vi "Find Transition.vi"(0 "State in":refnum<class "State.lvclass">, 5 "Target":string, 7 "Event":string, 9 "Type":string, 11 "error in (no error)":errorcluster) -> (4 "State thru":refnum<class "State.lvclass">, 6 "transIndex":i32, 8 "termination":bool, 15 "error out":errorcluster)   [LabVIEW 2015, in "State.lvclass"]
uses:
  State.lvclass
  Typedefs/Tosca-Event Type.ctl
  State.lvclass/State.ctl
  Termination/Termination.lvclass/Termination.ctl
  Timeout/Timeout.lvclass/Timeout.ctl
  Termination/Read Link to.vi
  Termination/Read Source.vi
  Termination/Read Type.vi
  Timeout/Read Link to.vi
  Timeout/Read Type.vi
  Timeout/Timeout.lvclass
  Termination/Termination.lvclass
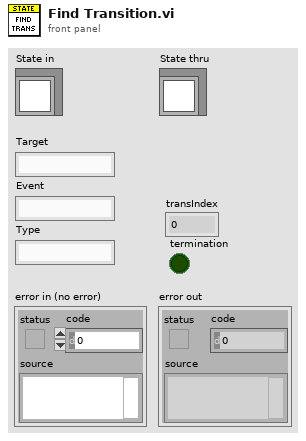
[diagram p1: front panel]
types:
  T1 = typedef "Tosca-Event Type.ctl" = enum16{"Normal", "CS+", "CS-"}
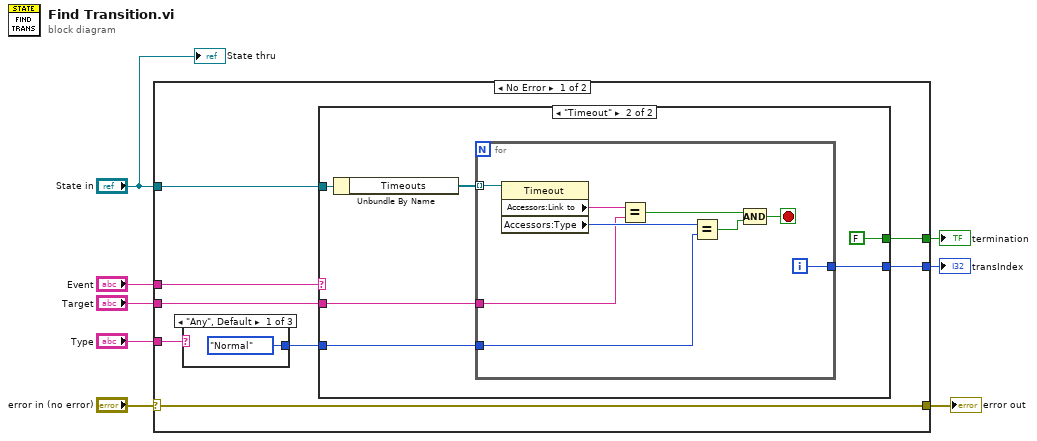
[diagram p0: block diagram]
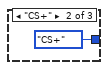
[diagram p2: hidden frame]
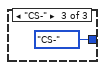
[diagram p3: hidden frame]
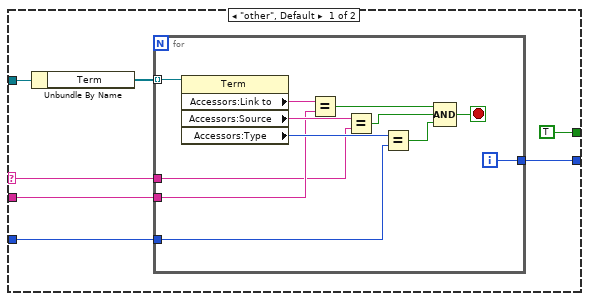
[diagram p4: hidden frame]
diagram:
  n1 = case shown="No Error" "error in (no error)" {
    selector: "error in (no error)" -> [w16 w54]
    tunnel: [w16 w54] -> w7
    tunnel: "State in" -> [w14 _]
    tunnel: "Type" -> [w10 _]
    tunnel: "Event" -> [w15 _]
    tunnel: "Target" -> [w13 _]
    tunnel: [w12 _] -> w3
    tunnel: [w11 _] -> w2
    frame No Error {
      n2 = case shown="\"Any\", Default" w10 {
        tunnel: [Tosca-Event_Type."Normal" ("Serialized.Type") Tosca-Event_Type."CS+" ("Serialized.Type") Tosca-Event_Type."CS-" ("Serialized.Type")] -> w9
        frame "Any", Default {
        }
        frame "CS+" {
        }
        frame "CS-" {
        }
      }
      n3 = case shown="\"Timeout\"" w15 {
        selector: w15 -> [w23 _]
        tunnel: w14 -> [w26 w44]
        tunnel: w13 -> [w24 w42]
        tunnel: [w22 w41] -> w12
        tunnel: [TRUE FALSE] -> w11
        tunnel: w9 -> [w20 w39]
        frame "other", Default {
          n4 = Unbundle By Name(w26) -> ("Term"=w25:refnum<class "Termination.lvclass">[])
          n5 = for {
            tunnel: w25 -> [w38] mode=indexing
            tunnel: w24 -> [w34]
            tunnel: w23 -> [w33]
            tunnel: [w29] -> w22
            tunnel: w20 -> [w27]
            i -> [w29]
            stop <- w28 stop-if-true
            n6 = property class="Term"(reference=w38) -> ("Accessors:Link to"=w37:string, "Accessors:Source"=w36:string, "Accessors:Type"=w35:T1)  [unwired: 1 in, 2 out]
            n7 = Equal?(x=w37, y=w34) -> (x = y?=w32:bool)
            n8 = Equal?(x=w36, y=w33) -> (x = y?=w31:bool)
            n9 = Equal?(x=w35, y=w27) -> (x = y?=w30:bool)
            n10 = Compound Arithmetic op=AND(w32, w31, w30) -> (w28:bool)
          }
        }
        frame "Timeout" {
          n11 = Unbundle By Name(w44) -> ("Timeouts"=w43:refnum<class "Timeout.lvclass">[])
          n12 = for {
            tunnel: w43 -> [w53] mode=indexing
            tunnel: w42 -> [w50]
            tunnel: [w47] -> w41
            tunnel: w39 -> [w45]
            i -> [w47]
            stop <- w46 stop-if-true
            n13 = property class="Timeout"(reference=w53) -> ("Accessors:Link to"=w52:string, "Accessors:Type"=w51:T1)  [unwired: 1 in, 2 out]
            n14 = Equal?(x=w52, y=w50) -> (x = y?=w49:bool)
            n15 = Equal?(x=w51, y=w45) -> (x = y?=w48:bool)
            n16 = Compound Arithmetic op=AND(w49, w48) -> (w46:bool)
          }
        }
      }
    }
    frame Error {
    }
  }
  "error out" <- w7
  "transIndex" <- w3
  "termination" <- w2
  "State thru" <- "State in"
